vi "GUI_DS-LaserFrontEndLogger.vi"() -> ()   [LabVIEW 2013]
uses:
  Shared/GUI_Template/GUI_master/tcp_new_data_event.ctl
  Shared/GUI_Template/GUI_master/tcp new data cluster.ctl
panel:
  out "XY Graph 3":cluster{timestamp[], dbl[]}[](graph)
  out "XY Graph 2":cluster{timestamp[], dbl[]}[](graph)
  out "XY Graph":cluster{timestamp[], dbl[]}(graph)
  in  "reading.var 7::1":dbl caption="Preamp1 power" min=-100000.0 max=100000.0
  in  "reading.var 6::1":dbl caption="Amp0 pulse energy" min=-100000.0 max=100000.0
  in  "reading.var 1::1":dbl caption="Regen pulse energy" min=-100000.0 max=100000.0
  in  "reading.var 3::1":dbl caption="XPW spectral width" min=-100000.0 max=100000.0
  in  "reading.var 2::1":dbl caption="XPW spec peak counts" min=-100000.0 max=100000.0
  out "tcp data event":T1
  in  "Refresh Button":bool
  out "XY Graph 5":T2(graph)
  in  "channel 2::2":dbl[](array[numeric]) caption="channel 1::2"
  in  "GUIdevice 2":string="DS-XPWspec"
  in  "channel 1::2":dbl[](array[numeric])
  in  "reading.var 8::1":dbl caption="XPW central wavelength" min=-100000.0 max=100000.0
  in  "refresh time (ms)":i32=500
  in  "reading.var 5::1":dbl caption="Amp0 input centriod Y" min=-100000.0 max=100000.0
  in  "reading.var 4::1":dbl caption="Amp0 input centriod x" min=-100000.0 max=100000.0
  in  "stop":bool
  in  "GUIdevice 1":string="DS-LaserFrontEndLogger"
  # "Laser front end logger"
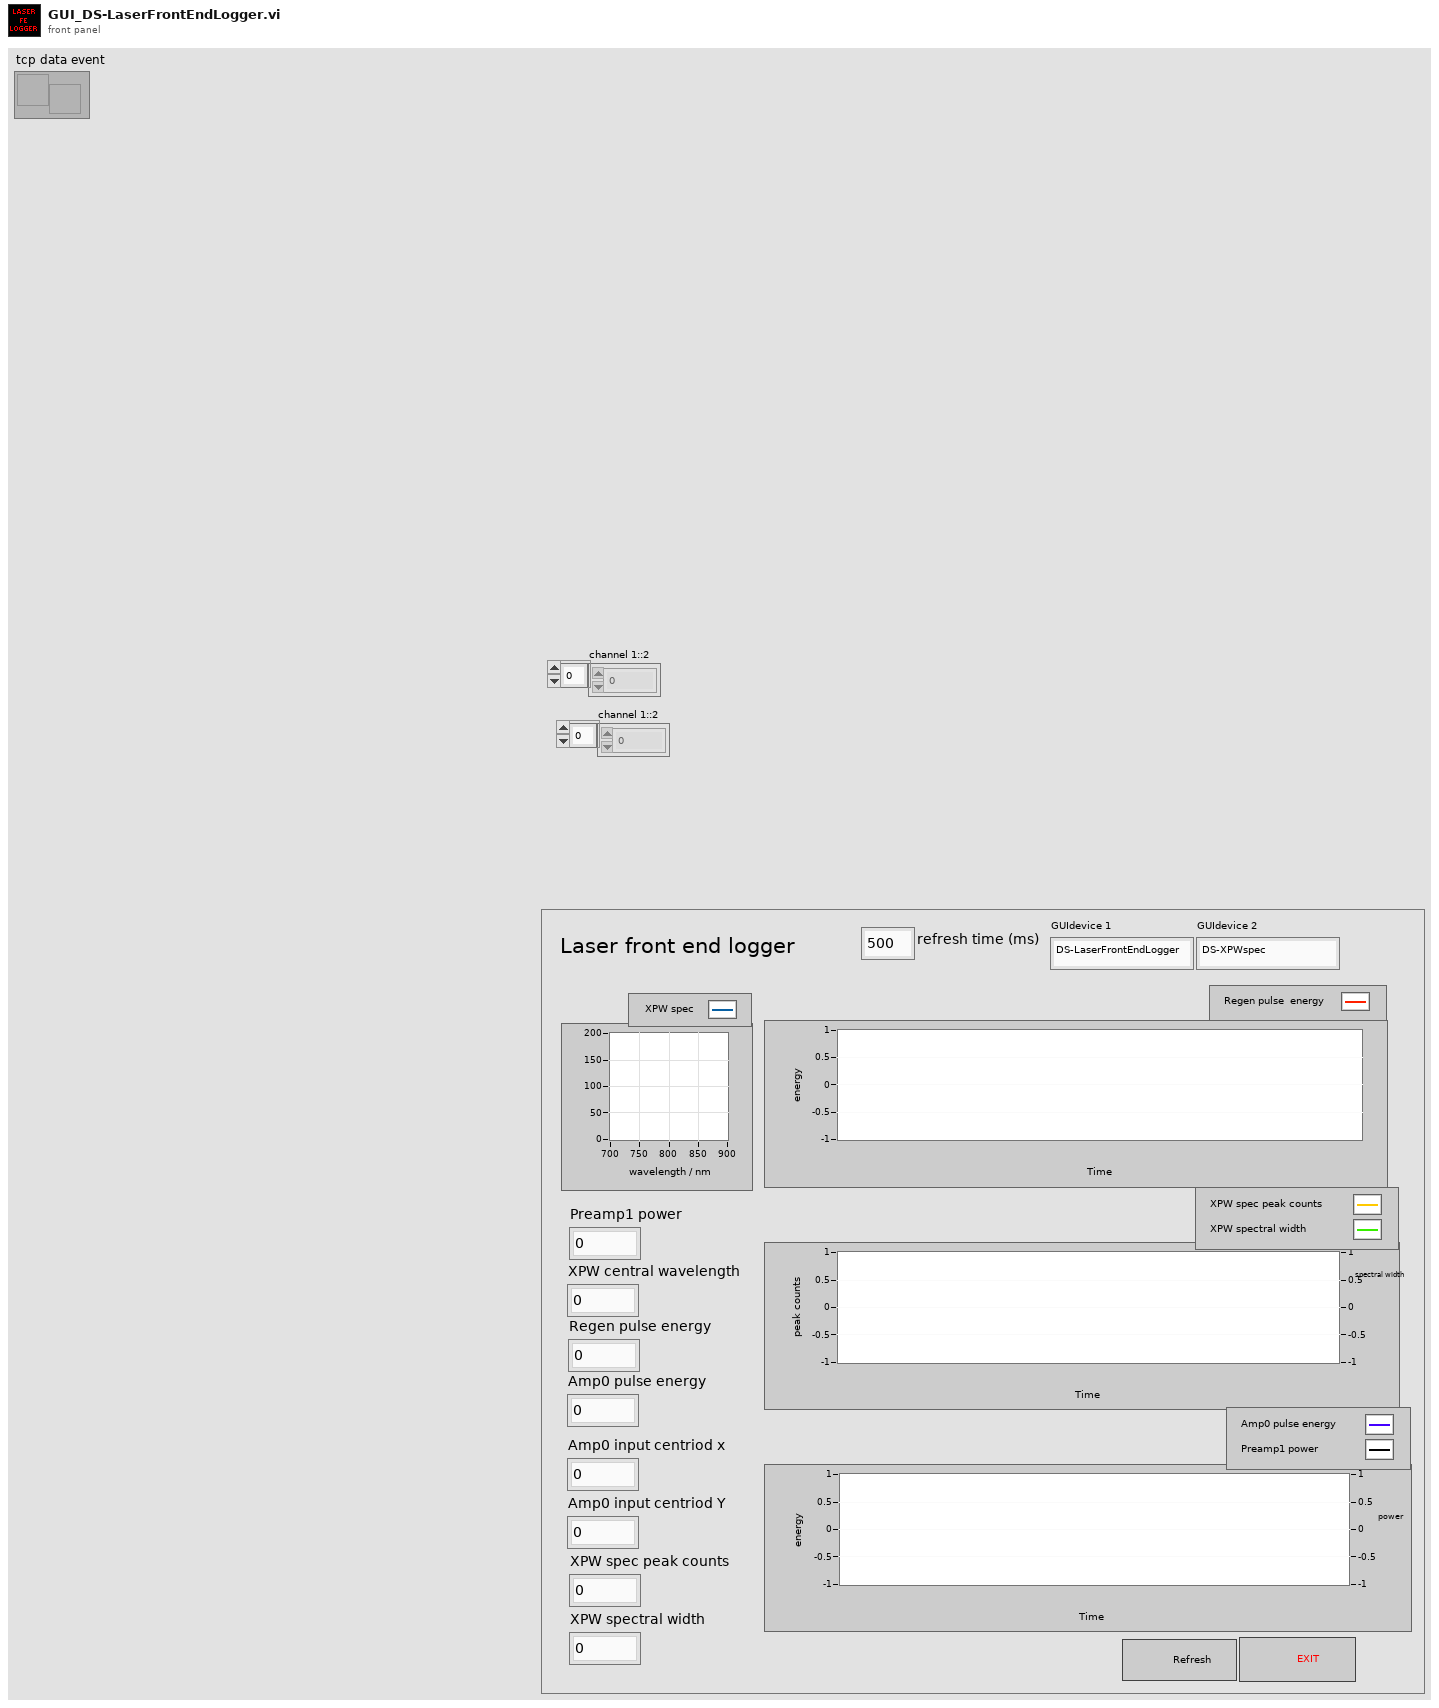
[diagram p1: front panel]
types:
  T1 = typedef "tcp_new_data_event.ctl" = refnum<user-event>
  T2 = cluster{"channel 1::2":dbl[], "channel 2::2":dbl[]}
  T3 = enum32{"invalid app kind", "Development System", "Run Time System", "Student Edition", "Embedded LabVIEW", "Evaluation", "Custom"}
  T4 = typedef "tcp new data cluster.ctl" = cluster{"EventEnum":enum16{"new data", "connection status update"}, "Device name":string}
  T5 = enum32{"Invalid", "Standard", "Closed", "Hidden", "Minimized", "Maximized"}
  T6 = cluster{"Core":cluster{"Current VI Reference":refnum<vi>, "Close Panel on Exit?":bool}, "Your Boolean data":bool, "Your string data":string, "SuperGUI":cluster{"STOP queue":refnum<queue>, "SuperGUI ref":refnum<vi>}, "Graph parameters":cluster{"Timestamp":dbl[], "variable 1":dbl[], "variable 2":dbl[], "variable 3":dbl[], "variable 7":dbl[], "variable 8":dbl[]}}
  T7 = cluster{"Timestamp":dbl[], "variable 1":dbl[], "variable 2":dbl[], "variable 3":dbl[], "variable 7":dbl[], "variable 8":dbl[]}
  T8 = cluster{"STOP queue":refnum<queue>, "SuperGUI ref":refnum<vi>}
  T9 = cluster{"Current VI Reference":refnum<vi>, "Close Panel on Exit?":bool}
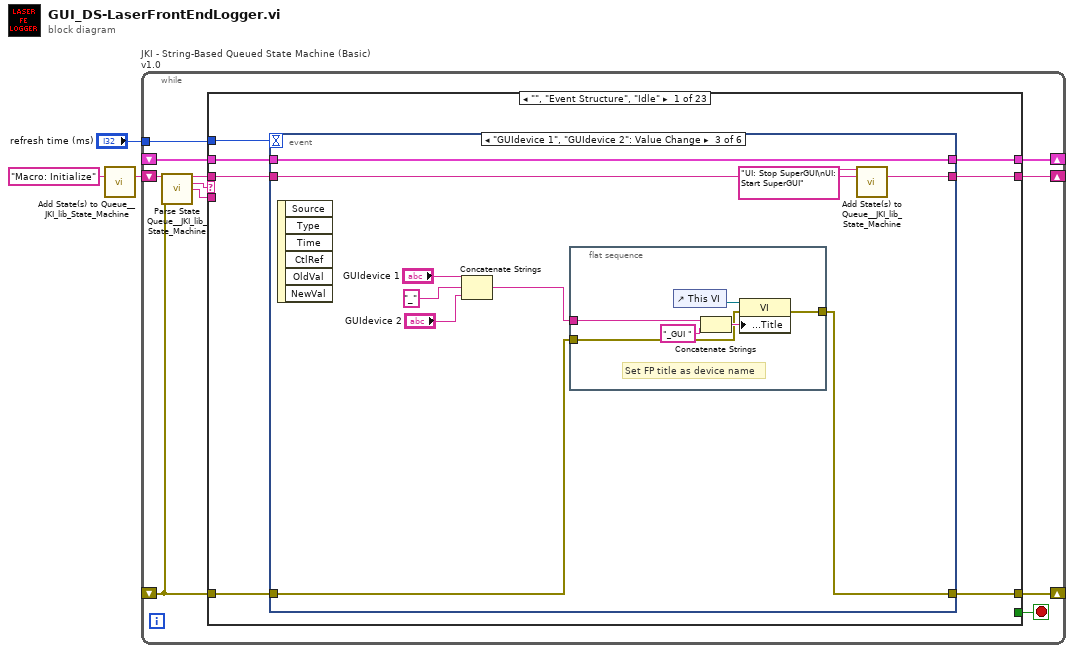
[diagram p0: block diagram]
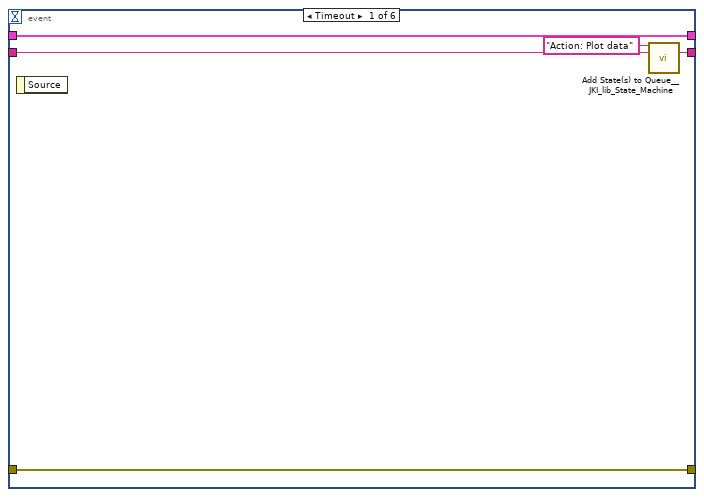
[diagram p2: hidden frame]
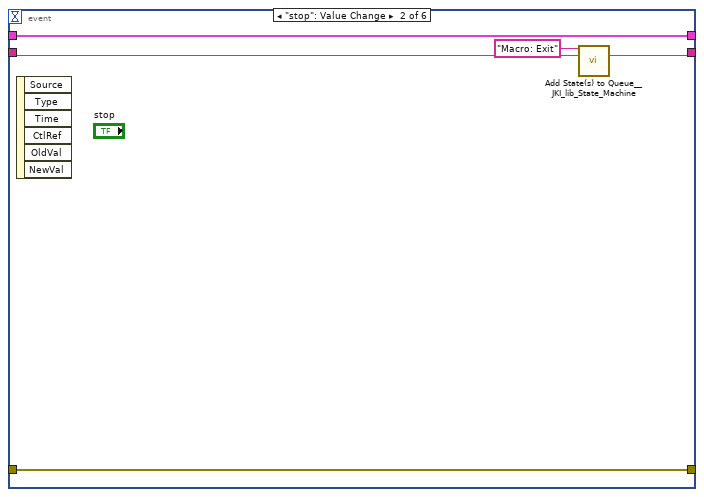
[diagram p3: hidden frame]
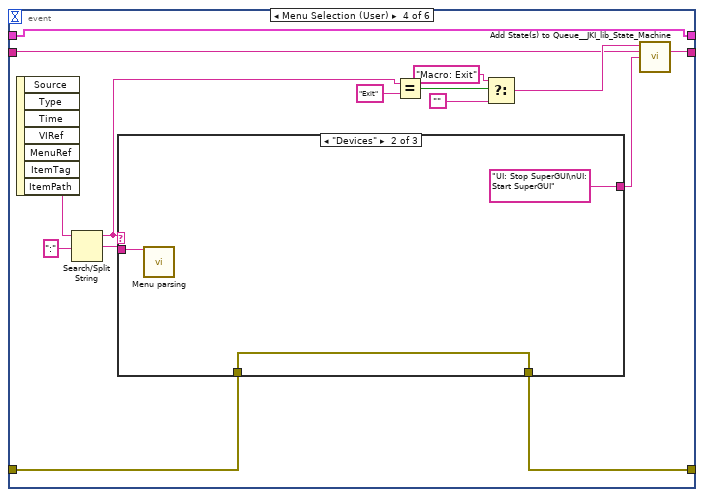
[diagram p4: hidden frame]
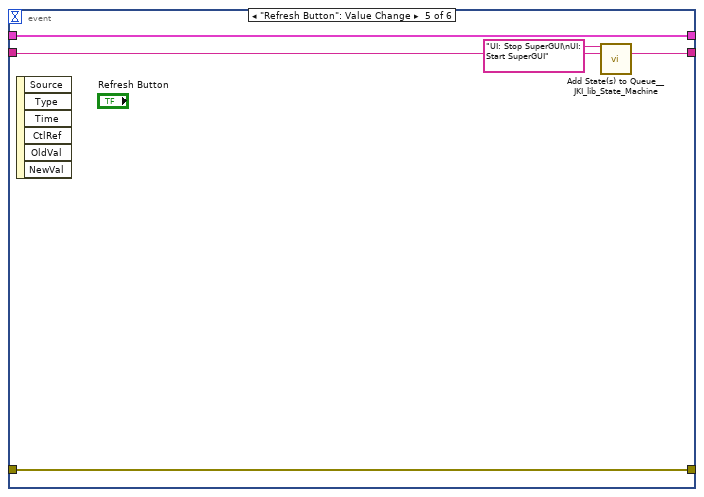
[diagram p7: hidden frame]
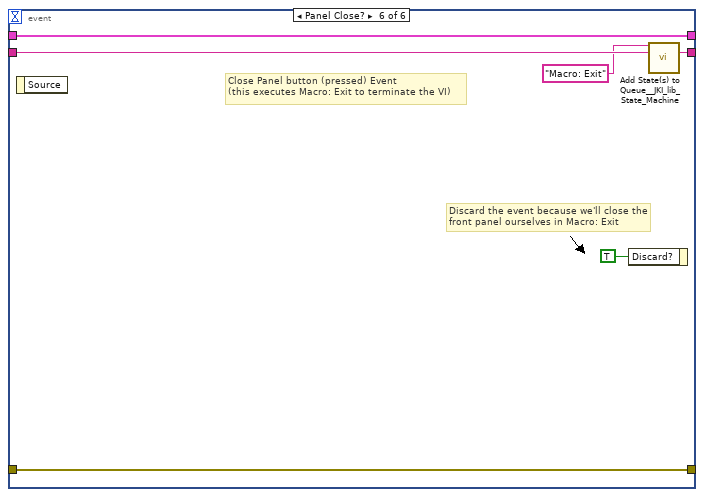
[diagram p8: hidden frame]
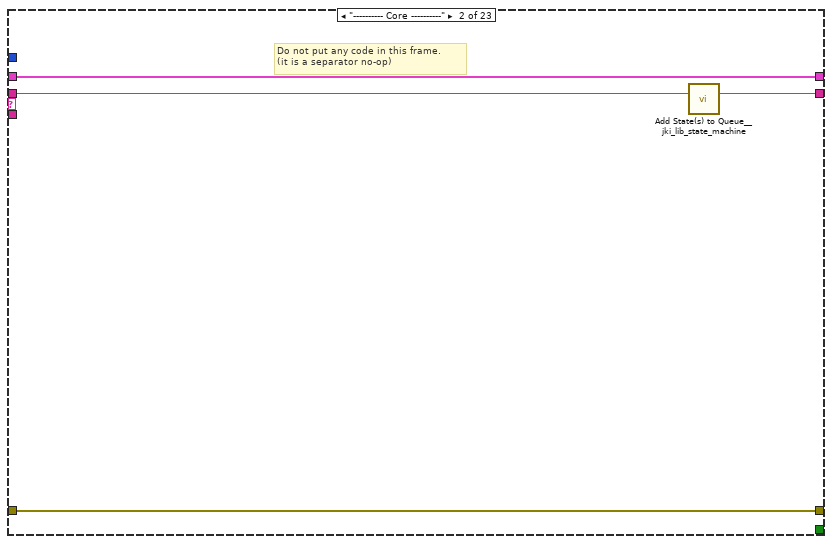
[diagram p9: hidden frame]
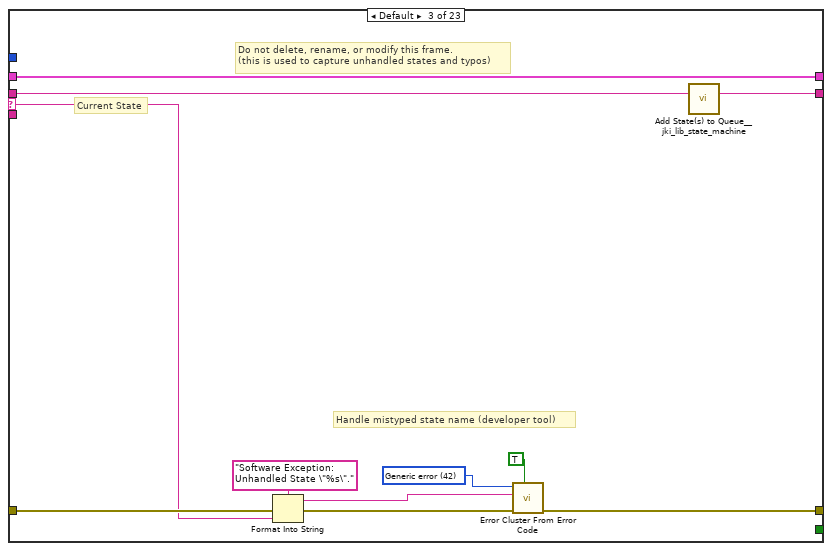
[diagram p10: hidden frame]
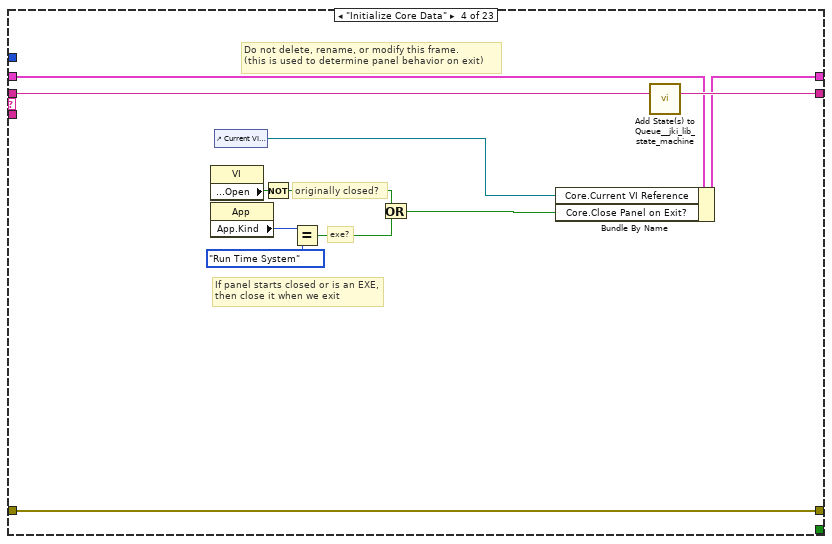
[diagram p11: hidden frame]
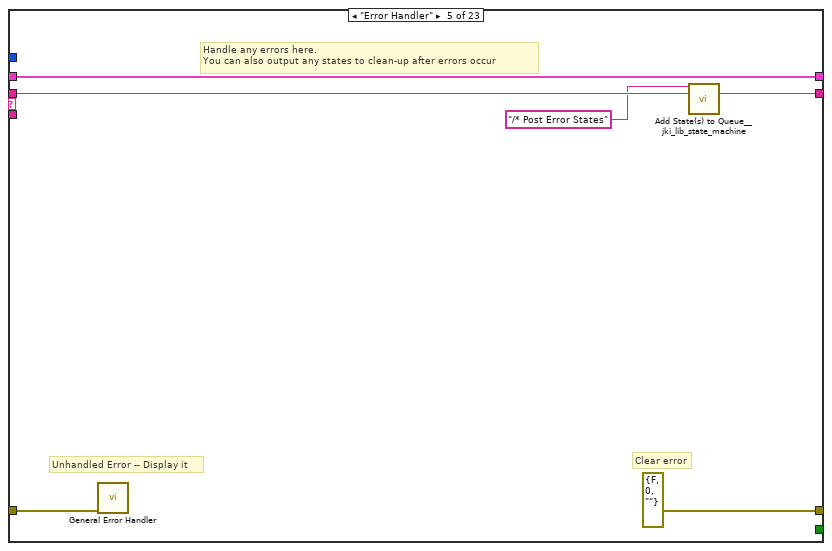
[diagram p12: hidden frame]
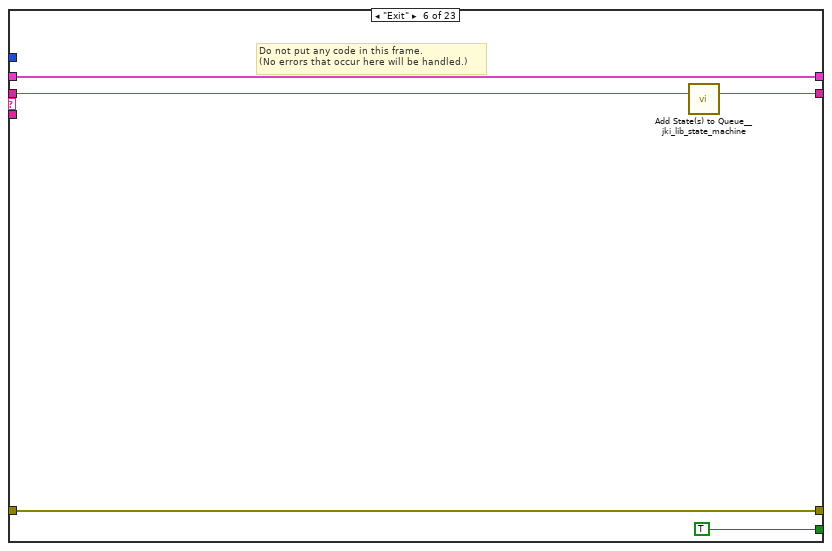
[diagram p13: hidden frame]
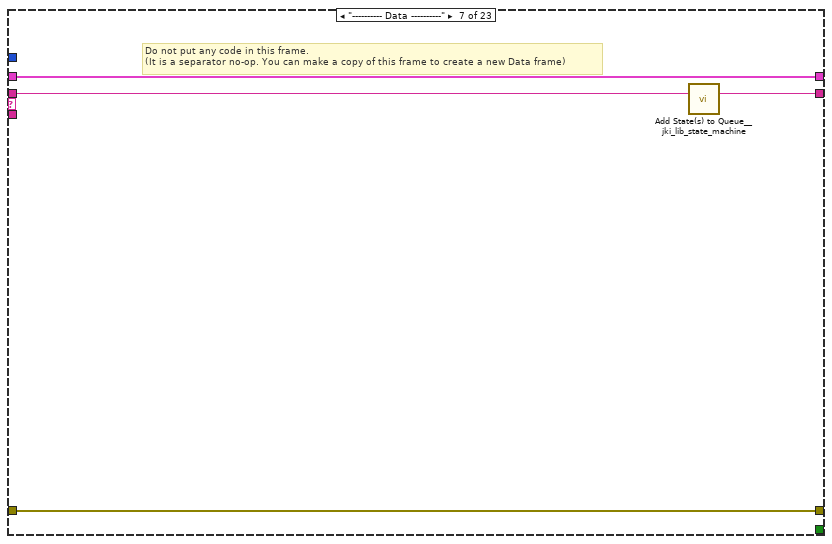
[diagram p14: hidden frame]
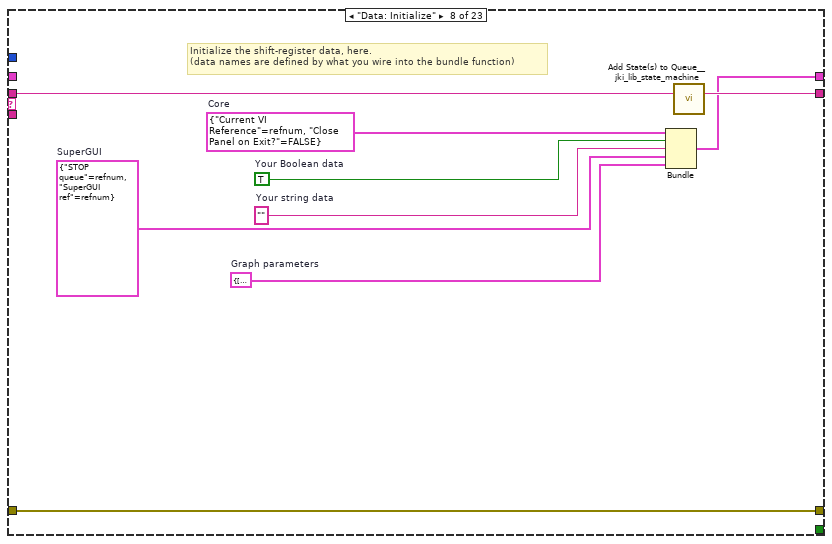
[diagram p15: hidden frame]
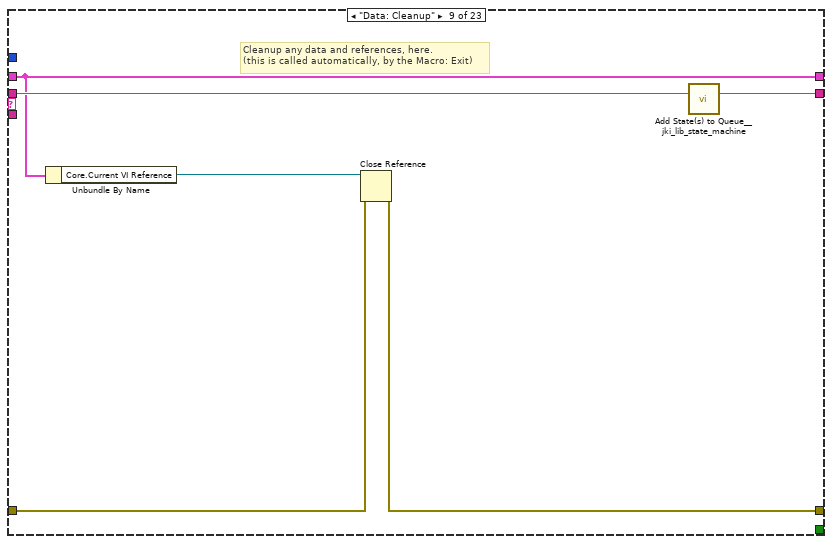
[diagram p16: hidden frame]
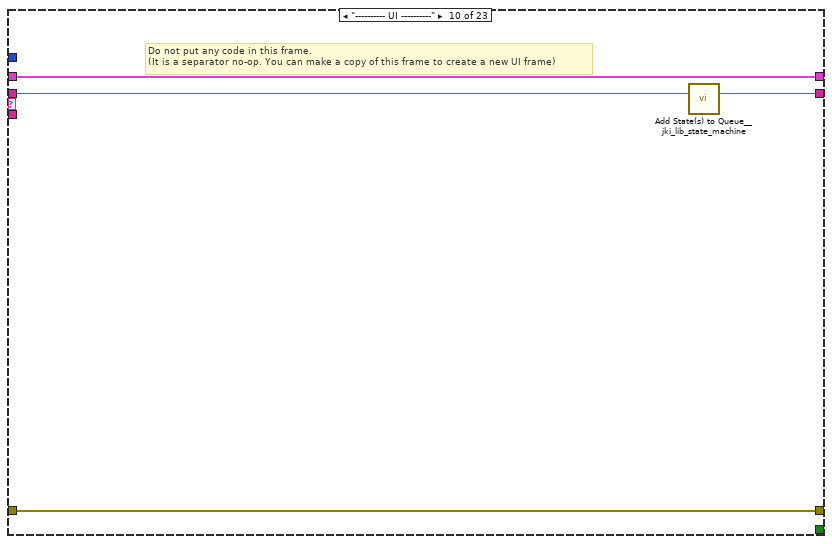
[diagram p17: hidden frame]
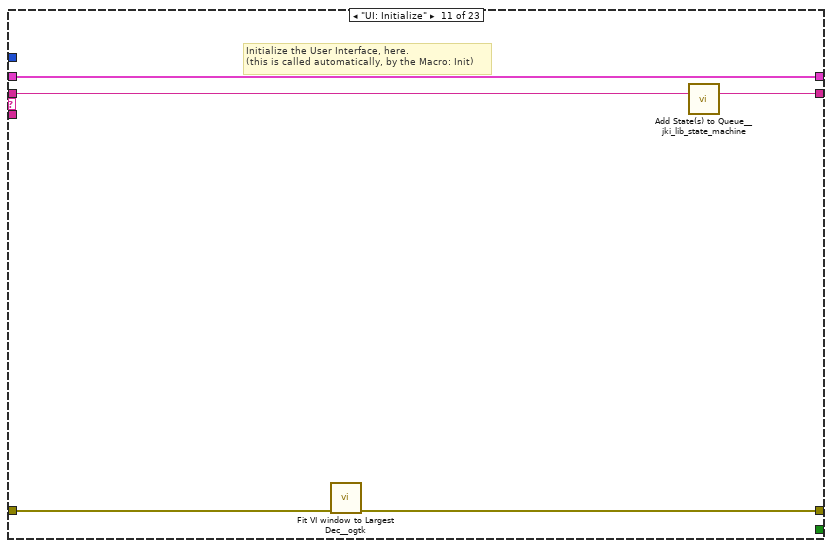
[diagram p18: hidden frame]
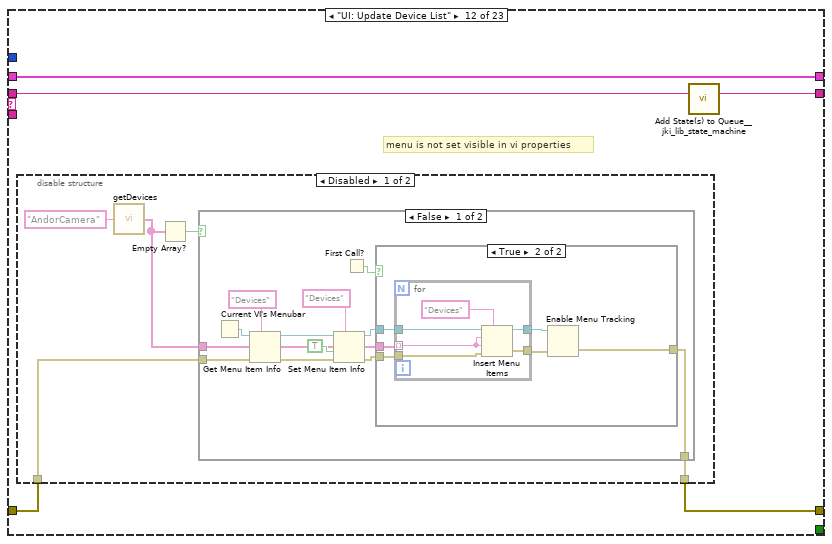
[diagram p19: hidden frame]
diagram:
  n1 = call <vilib>:"Add State(s) to Queue__JKI_lib_State_Machine.vi"("State(s) in (\"\")"="Macro: Initialize") -> ("States Out"=w3:string)  [unwired: 14 in]
  n2 = while "JKI - String-Based Queued State Machine (Basic) v1.0" {
    shift-right: [w7] -> _
    shift-left: _ -> [w6]
    shift-right: [w10] -> _
    shift-left: _ -> [w5]
    shift-right: [w9] -> _
    shift-left: w3 -> [w11]
    tunnel: "refresh time (ms)" -> [w4]
    stop <- w8 stop-if-true
    n3 = call <vilib>:"Parse State Queue__JKI_lib_State_Machine.vi"("State Queue"=w11, "Error In (no error)"=w5) -> ("Remaining States"=w13:string, "Current State"=w14:string, "Arguments"=w12:string)  [unwired: 11 in]
    n4 = case shown="\"\", \"Event Structure\", \"Idle\"" w14 {
      selector: w14 -> [_ _ w83 _ _ _ _ _ _ _ _ _ _ _ _ _ _ _ _ _ _ _ _]
      tunnel: w13 -> [w21 w82 w87 w105 w111 w116 w120 w129 w135 w139 w144 w149 w187 w221 w229 w235 w246 w272 w277 w287 w291 w329 w376]
      tunnel: w12 -> [_ _ _ _ _ _ _ _ _ _ _ _ _ _ _ w230 w240 _ _ _ _ _ _]
      tunnel: w6 -> [w19 w79 w85 w96 w108 w114 w117 _ w130 w136 w142 w147 w185 w212 w224 w233 w242 w269 w274 w284 w288 w299 w373]
      tunnel: [w18 w80 w89 w102 errorcluster {"status"=FALSE, "code"=0, "source"=""} ("error out") w113 w118 w126 w131 w137 w140 w145 w182 w205 w222 w231 w243 w270 w275 w285 w289 w327 w374] -> w10
      tunnel: w5 -> [w17 w80 w88 w102 w107 w113 w118 w126 w132 w137 w141 w146 w183 w206 w223 w232 w244 w270 w275 w285 w289 w327 w374]
      tunnel: [w20 w81 w86 w104 w110 w115 w119 w128 w134 w138 w143 w148 w186 w220 w228 w234 w245 w271 w276 w286 w290 w328 w375] -> w9
      tunnel: [_ _ _ _ _ TRUE _ _ _ _ _ _ _ _ _ _ _ _ _ _ _ _ _] -> w8
      tunnel: [w16 w79 w85 w103 w108 w114 w117 w127 w130 w136 w142 w147 w185 w211 w224 w233 w242 w269 w274 w284 w288 w298 w373] -> w7
      tunnel: w4 -> [w15 _ _ _ _ _ _ _ _ _ _ _ _ _ _ _ _ _ _ _ _ _ _]
      frame "", "Event Structure", "Idle" {
        n5 = event shown="[2] \"GUIdevice 1\", \"GUIdevice 2\": Value Change" {
          selector: _ -> [_ _ _ _ _ _]
          dyn-events: _ -> [_ _ _ _ _ _]
          timeout: w15 -> [_ _ _ _ _ _]
          tunnel: w21 -> [w26 w29 w40 w56 w70 w78]
          tunnel: [w25 w28 w39 w55 w69 w77] -> w20
          tunnel: w19 -> [w23 w31 w41 w62 w72 w75]
          tunnel: [w24 w30 w33 w49 w71 w76] -> w18
          tunnel: w17 -> [w24 w30 w34 w50 w71 w76]
          tunnel: [w23 w31 w41 w62 w72 w75] -> w16
          event Timeout {
            n6 = event-data() -> ()  [unwired: 1 in, 1 out]
            n7 = call <vilib>:"Add State(s) to Queue__JKI_lib_State_Machine.vi"("State(s) in Front (\"\")"="Action: Plot data" ("State(s) in Front (\"\")"), "State(s) in (\"\")"=w26) -> ("States Out"=w25:string)  [unwired: 13 in]
          }
          event "stop": Value Change {
            n8 = event-data() -> ()  [unwired: 1 in, 6 out]
            n9 = call <vilib>:"Add State(s) to Queue__JKI_lib_State_Machine.vi"("State(s) in Front (\"\")"="Macro: Exit", "State(s) in (\"\")"=w29) -> ("States Out"=w28:string)  [unwired: 13 in]
          }
          event "GUIdevice 1", "GUIdevice 2": Value Change {
            n10 = event-data() -> ()  [unwired: 1 in, 6 out]
            n11 = Concatenate Strings("GUIdevice 1", "_", "GUIdevice 2") -> (w35:string)
            n12 = flat-sequence {
              tunnel: [w44] -> w33
              tunnel: w34 -> [w43]
              tunnel: w35 -> [w42]
              frame #0 {
                # "Set FP title as device name"
                n13 = control-ref of="This VI"() -> (w47:refnum<vi>)
                n14 = Concatenate Strings(w42, "_GUI ") -> (w46:string)
                n15 = property class="VI"(reference=w47, error in=w43, "Front Panel.Title"=w46) -> (error out=w44:errorcluster)  [unwired: 1 out]
              }
            }
            n16 = call <vilib>:"Add State(s) to Queue__JKI_lib_State_Machine.vi"("State(s) in Front (\"\")"="UI: Stop SuperGUI\nUI: Start SuperGUI", "State(s) in (\"\")"=w40) -> ("States Out"=w39:string)  [unwired: 13 in]
          }
          event Menu Selection (User) {
            n17 = event-data() -> ("ItemPath"=w52:string)  [unwired: 1 in, 6 out]
            n18 = Search/Split String(string=w52, search string/char (-)=":") -> (substring before match=w48:string, match + rest of string=w51:string)  [unwired: 1 in, 1 out]
            n19 = case shown="\"Devices\"" w48 {
              tunnel: w51 -> [_ w66 _]
              tunnel: w50 -> [w63 w64 w67]
              tunnel: [w63 w64 w67] -> w49
              tunnel: [_ "UI: Stop SuperGUI\nUI: Start SuperGUI" _] -> w54
              frame "", Default {
              }
              frame "Devices" {
                n20 = call "Menu parsing.vi"("ItemPath"=w66) -> ()  [unwired: 9 in, 2 out]
              }
              frame "Exit" {
              }
            }
            n21 = Equal?(x=w48, y="Exit") -> (x = y?=w60:bool)
            n22 = Select(t="Macro: Exit", s=w60, f="") -> (s? t:f=w57:string)
            n23 = call <vilib>:"Add State(s) to Queue__JKI_lib_State_Machine.vi"("State(s) in Front (\"\")"=w57, "State(s) in (\"\")"=w56, "State(s) at Back (\"\")"=w54) -> ("States Out"=w55:string)  [unwired: 12 in]
          }
          event "Refresh Button": Value Change {
            n24 = event-data() -> ()  [unwired: 1 in, 6 out]
            n25 = call <vilib>:"Add State(s) to Queue__JKI_lib_State_Machine.vi"("State(s) in Front (\"\")"="UI: Stop SuperGUI\nUI: Start SuperGUI", "State(s) in (\"\")"=w70) -> ("States Out"=w69:string)  [unwired: 13 in]
          }
          event Panel Close? {
            # "Discard the event because we'll close the front panel ourselves in Macro: Exit"
            # "Close Panel button (pressed) Event\n(this executes Macro: Exit to terminate the VI)"
            n26 = event-data() -> ()  [unwired: 1 in, 1 out]
            n27 = event-data("Discard?"=TRUE) -> ()  [unwired: 1 in, 1 out]
            n28 = call <vilib>:"Add State(s) to Queue__JKI_lib_State_Machine.vi"("State(s) in Front (\"\")"="Macro: Exit", "State(s) in (\"\")"=w78) -> ("States Out"=w77:string)  [unwired: 13 in]
          }
        }
      }
      frame "---------- Core ----------" {
        # "Do not put any code in this frame.\n(it is a separator no-op)"
        n29 = call <vilib>:"Add State(s) to Queue__jki_lib_state_machine.vi"("State(s) in (\"\")"=w82) -> ("States Out"=w81:string)  [unwired: 14 in]
      }
      frame Default {
        w92 = 42 items=["No error", "Argument error", "Memory is full", "Out of zone", "End of file", "File already open", "Generic file I/O error", "File not found", "File permission error", "Disk is full", "Duplicate path", "Too many files open", "System feature not enabled", "Resource file not found", "Cannot add resource", "Resource not found", "Image not found", "Image memory error", "Pen does not exist", "Config type invalid", "Config token not found", "Config parse error", "Config memory error", "Bad external code format", "Bad external code offset", "External code not present", "Null window", "Destroy window error", "Null menu", "Print aborted", "Bad print record", "Print driver error", "Windows error during printing", "Memory error during printing", "Print dialog error", "Generic print error", "Invalid device refnum", "Device not found", "Device parameter error", "Device unit error", "Cannot open device", "Device call aborted", "Generic error", "Cancelled by user", "Object ID too low", "Object ID too high", "Object not in heap", "Unknown heap", "Unknown object (invalid DefProc)", "Unknown object (DefProc not in table)", "Message out of range", "Invalid (null) method", "Unknown message", "Manager call not supported", "Bad address", "Network operation in progress", "Network operation timed out", "Connection is busy", "Network attribute not supported", "Network error", "Address in use", "System out of memory", "Connection aborted", "Connection refused", "Not connected", "Already connected", "Connection closed", "Initialization error (interapplication manager)", "Bad occurrence", "Wait on unbound occurrence handler", "Occurrence queue overflow", "Datalog type conflict", "Unused", "Unrecognized type (interapplication manager)", "Memory corrupt", "Failed to make temporary DLL", "Old CIN version", "Drag socket not found", "Failed to load drop-object", "Failed to register OLE object", "Failed to release OLE object", "Format specifier type mismatch", "Unknown format specifier", "Too few format specifiers", "Too many format specifiers", "Scan failed", "Newer CIN version", "Error converting to variant", "Runtime menu error", "Password tampered", "Variant attribute not found", "Incompatible variant data type", "Event data is not available", "Event Store is not present", "Occurrence is not found", "Event Queue is not created", "Event info is not available", "Refnum passed is NULL", "Error retrieving Class GUID", "Error retrieving CoClass GUID", "Error retrieving TypeLib GUID.", "Bad built application magic bytes.", "Specific driver is different from the specific driver associated with the Logical Name.", "There is no session opened to the class driver.", "Max Error", "MAX - Error with config objects", "MAX - Error loading configuration", "MAX - Group not supported"]
        # "Current State"
        # "Do not delete, rename, or modify this frame.\n(this is used to capture unhandled states and typos)"
        # "Handle mistyped state name (developer tool)"
        n30 = Format Into String(format string="Software Exception: Unhandled State \"%s\"." ("message"), error in=w88, w83) -> (resulting string=w91:string, error out=w90:errorcluster)  [unwired: 1 in]
        n31 = call <vilib>:"Error Cluster From Error Code.vi"("show call chain? (False)"=TRUE, "error in (no error)"=w90, "error message (\"\")"=w91, "error code (0)"=w92) -> ("error out"=w89:errorcluster)  [unwired: 5 in]
        n32 = call <vilib>:"Add State(s) to Queue__jki_lib_state_machine.vi"("State(s) in (\"\")"=w87) -> ("States Out"=w86:string)  [unwired: 14 in]
      }
      frame "Initialize Core Data" {
        # "Do not delete, rename, or modify this frame.\n(this is used to determine panel behavior on exit)"
        # "originally closed?"
        # "exe?"
        # "If panel starts closed or is an EXE, then close it when we exit"
        n33 = property class="VI"() -> ("Front Panel.Open"=w101:bool)  [unwired: 2 in, 2 out]
        n34 = property class="App"() -> ("App.Kind"=w100:T3)  [unwired: 2 in, 2 out]
        n35 = control-ref of="Current VI Reference"() -> (w94:refnum<vi>)
        n36 = Not(x=w101) -> (.not. x?=w98:bool)
        n37 = Equal?(x=w100, y=T3."Run Time System" ("Application:Kind")) -> (x = y?=w97:bool)
        n38 = Or(x=w98, y=w97) -> (x .or. y?=w95:bool)
        n39 = Bundle By Name(cluster=w96, "Core.Current VI Reference"=w94, "Core.Close Panel on Exit?"=w95) -> (w103:T6)
        n40 = call <vilib>:"Add State(s) to Queue__jki_lib_state_machine.vi"("State(s) in (\"\")"=w105) -> ("States Out"=w104:string)  [unwired: 14 in]
      }
      frame "Error Handler" {
        # "Unhandled Error -- Display it"
        # "Handle any errors here.\nYou can also output any states to clean-up after errors occur"
        # "Clear error"
        n41 = call <vilib>:"General Error Handler.vi"("error in (no error)"=w107) -> ()  [unwired: 10 in, 5 out]
        n42 = call <vilib>:"Add State(s) to Queue__jki_lib_state_machine.vi"("State(s) in Front (\"\")"="/* Post Error States", "State(s) in (\"\")"=w111) -> ("States Out"=w110:string)  [unwired: 13 in]
      }
      frame "Exit" {
        # "Do not put any code in this frame.\n(No errors that occur here will be handled.)"
        n43 = call <vilib>:"Add State(s) to Queue__jki_lib_state_machine.vi"("State(s) in (\"\")"=w116) -> ("States Out"=w115:string)  [unwired: 14 in]
      }
      frame "---------- Data ----------" {
        # "Do not put any code in this frame.\n(It is a separator no-op. You can make a copy of this frame to create a new Data frame)"
        n44 = call <vilib>:"Add State(s) to Queue__jki_lib_state_machine.vi"("State(s) in (\"\")"=w120) -> ("States Out"=w119:string)  [unwired: 14 in]
      }
      frame "Data: Initialize" {
        w121 = T7 {"Timestamp"=[], "variable 1"=[], "variable 2"=[], "variable 3"=[], "variable 7"=[], "variable 8"=[]}  # Graph parameters
        w122 = T8 {"STOP queue"=refnum, "SuperGUI ref"=refnum}  # SuperGUI
        w123 = T9 {"Current VI Reference"=refnum, "Close Panel on Exit?"=FALSE}  # Core
        w125 = TRUE  # Your Boolean data
        w124 = ""  # Your string data
        # "Initialize the shift-register data, here.\n(data names are defined by what you wire into the bundle function)"
        n45 = Bundle("Core"=w123, "Your Boolean data"=w125, "Your string data"=w124, "SuperGUI"=w122, "Graph parameters"=w121) -> (w127:T6)  [unwired: 1 in]
        n46 = call <vilib>:"Add State(s) to Queue__jki_lib_state_machine.vi"("State(s) in (\"\")"=w129) -> ("States Out"=w128:string)  [unwired: 14 in]
      }
      frame "Data: Cleanup" {
        # "Cleanup any data and references, here.\n(this is called automatically, by the Macro: Exit)"
        n47 = Unbundle By Name(w130) -> ("Core.Current VI Reference"=w133:refnum<vi>)
        n48 = Close Reference(reference=w133, error in (no error)=w132) -> (error out=w131:errorcluster)
        n49 = call <vilib>:"Add State(s) to Queue__jki_lib_state_machine.vi"("State(s) in (\"\")"=w135) -> ("States Out"=w134:string)  [unwired: 14 in]
      }
      frame "---------- UI ----------" {
        # "Do not put any code in this frame.\n(It is a separator no-op. You can make a copy of this frame to create a new UI frame)"
        n50 = call <vilib>:"Add State(s) to Queue__jki_lib_state_machine.vi"("State(s) in (\"\")"=w139) -> ("States Out"=w138:string)  [unwired: 14 in]
      }
      frame "UI: Initialize" {
        # "Initialize the User Interface, here.\n(this is called automatically, by the Macro: Init)"
        n51 = call <userlib>:"Fit VI window to Largest Dec__ogtk.vi"("error in (no error)"=w141) -> ("error out"=w140:errorcluster)  [unwired: 5 in, 1 out]
        n52 = call <vilib>:"Add State(s) to Queue__jki_lib_state_machine.vi"("State(s) in (\"\")"=w144) -> ("States Out"=w143:string)  [unwired: 14 in]
      }
      frame "UI: Update Device List" {
        # "menu is not set visible in vi properties"
        n53 = disable-structure shown="Disabled" {
          disable-tunnel: w146 -> [w154 w181]
          disable-tunnel: [w152 w181] -> w145
          frame Disabled {
            n54 = call "getDevices.vi"("Device Class"="AndorCamera") -> ("All Devices"=w150:string[])
            n55 = Empty Array?(array=w150) -> (empty?=w151:bool)
            n56 = case shown="False" w151 {
              tunnel: w154 -> [w157 w180]
              tunnel: [w156 w180] -> w152
              tunnel: w150 -> [w155 _]
              frame False {
                n57 = Current VI's Menubar() -> (w160:refnum<k9>)
                n58 = Get Menu Item Info(7:"Devices" ("item tag"), 8:w157, 11:w160) -> (0:w166:errorcluster, 3:w162:refnum<k9>)  [unwired: 5 out]
                n59 = Set Menu Item Info(7:"Devices" ("item tag"), 8:w166, 9:TRUE ("enabled"), 11:w162) -> (0:w165:errorcluster, 3:w164:refnum<k9>)  [unwired: 3 in]
                n60 = First Call?() -> (First Call?: T/F=w158:bool)
                n61 = case shown="True" w158 {
                  tunnel: w164 -> [_ w172]
                  tunnel: w155 -> [_ w171]
                  tunnel: w165 -> [w167 w169]
                  tunnel: [w167 w168] -> w156
                  frame False {
                  }
                  frame True {
                    n62 = for {
                      tunnel: [w179] -> w173
                      tunnel: w171 -> [w177] mode=indexing
                      tunnel: w172 -> [w176]
                      tunnel: [w175] -> w170
                      tunnel: w169 -> [w174]
                      n63 = Insert Menu Items(5:"Devices" ("menu tag"), 6:w174, 7:w177, 8:w177, 9:w176) -> (0:w175:errorcluster, 3:w179:refnum<k9>)  [unwired: 1 in, 1 out]
                    }
                    n64 = Enable Menu Tracking(2:w170, 4:w173) -> (0:w168:errorcluster)  [unwired: 1 in, 1 out]
                  }
                }
              }
              frame True {
              }
            }
          }
          frame Enabled {
          }
        }
        n65 = call <vilib>:"Add State(s) to Queue__jki_lib_state_machine.vi"("State(s) in (\"\")"=w149) -> ("States Out"=w148:string)  [unwired: 14 in]
      }
      frame "UI: Get Device Name" {
        n66 = First Call?() -> (First Call?: T/F=w184:bool)
        n67 = case shown="True" w184 {
          tunnel: w183 -> [w188 w190]
          tunnel: [w188 w189] -> w182
          frame False {
          }
          frame True {
            n68 = disable-structure "Get Device name from control for vi mode\nand command line arg for exe" shown="RUN_TIME_ENGINE==True" {
              disable-tunnel: w190 -> [w191 w193]
              disable-tunnel: [w191 w192] -> w189
              frame condition #0 (active) {
              }
              frame condition #1 {
                n69 = control-ref of="This Application"() -> (w201:refnum<vi>)
                n70 = property class="App"(reference=w201) -> ("App.Args"=w200:string[])  [unwired: 1 in, 2 out]
                n71 = Index Array(array=w200, index #1=1 ("index")) -> (element #1=w194:string)  [unwired: 2 in, 2 out]
                n72 = Empty String/Path?(string/path=w194) -> (empty?=w198:bool)
                n73 = control-ref of="This VI"() -> (w197:refnum<vi>)
                n74 = case shown="False" w198 {
                  frame False {
                  }
                  frame True {
                  }
                }
                n75 = Concatenate Strings(w194, "_GUI ") -> (w196:string)
                n76 = property class="VI"(reference=w197, error in=w193, "Front Panel.Title"=w196) -> (error out=w192:errorcluster)  [unwired: 1 out]
              }
            }
          }
        }
        n77 = call <vilib>:"Add State(s) to Queue__jki_lib_state_machine.vi"("State(s) in (\"\")"=w187) -> ("States Out"=w186:string)  [unwired: 14 in]
      }
      frame "UI: Start SuperGUI" {
        # "create stop queue for supergui and its clones"
        # "x100 abort will be dependent on caller VI\nx80 abort will be independent of caller vi, this will abort vi when labview is closed."
        # "Start SuperGUI asynchronous way"
        n78 = vi-ref "GUI_Master_subvi_reentrant_queues.vi"() -> (w204:refnum<vi>)
        n79 = property class="VI"(reference=w204) -> ("Path"=w203:path)  [unwired: 1 in, 2 out]
        n80 = Create User Event(user event datatype=T4 {"EventEnum"=enum."new data", "Device name"="Device name"} ("New Event"), error in=w206) -> (user event=w207:refnum<user-event>, error out=w213:errorcluster)
        "tcp data event" <- w207
        n81 = control-ref of="This Application"() -> (w210:refnum<vi>)
        n82 = control-ref of="This VI"() -> (w209:refnum<vi>)
        n83 = Open VI Reference(type specifier VI Refnum (for type only)=refnum<vi> refnum, vi path=w203, options=256) -> (vi reference=w219:refnum<vi>, error out=w218:errorcluster)  [unwired: 3 in]
        n84 = register-events(w207) -> ()  [unwired: 2 in, 2 out]
        n85 = call "supergui create stop queue.vi"() -> ("STOP Queue out"=w215:refnum<queue>)  [unwired: 11 in]
        n86 = Current VI's Menubar() -> (w208:refnum<k9>)
        n87 = call-by-ref "Start Asynchronous Call"(reference=w219, error in=w218, "STOP Queue in"=w215, "This Application"=w210, 8:"error in (no error)"=w213, "tcp data event"=w207, "Caller menu reference"=w208, "Caller VI ref"=w209) -> (reference out=w202:refnum<vi>, error out=w205:errorcluster)  [unwired: 5 in, 1 out]
        n88 = Bundle By Name(cluster=w212, "SuperGUI.SuperGUI ref"=w202, "SuperGUI.STOP queue"=w215) -> (w211:T6)
        n89 = call <vilib>:"Add State(s) to Queue__jki_lib_state_machine.vi"("State(s) in (\"\")"=w221) -> ("States Out"=w220:string)  [unwired: 14 in]
      }
      frame "UI: Stop SuperGUI" {
        # "Stop Supergui Clone and wait until it exit properly"
        n90 = Unbundle By Name(w224) -> ("SuperGUI.SuperGUI ref"=w226:refnum<vi>, "SuperGUI.STOP queue"=w225:refnum<queue>)
        n91 = Release Queue(queue=w225, error in (no error)=w223) -> (error out=w227:errorcluster)  [unwired: 1 in, 2 out]
        n92 = call-by-ref "Wait On Asynchronous Call"(reference=w226, error in=w227) -> ("error out"=w222:errorcluster)  [unwired: 11 in, 2 out]
        n93 = call <vilib>:"Add State(s) to Queue__jki_lib_state_machine.vi"("State(s) in (\"\")"=w229) -> ("States Out"=w228:string)  [unwired: 14 in]
      }
      frame "UI: Cursor Set" {
        # "Argument"
        # "Set and Unset Cursor Busy.\n(Usage: \"UI: Cursor Set >> Busy|Idle\")"
        n94 = case shown="\"Idle\", Default" w230 {
          tunnel: w232 -> [w237 w239]
          tunnel: [w236 w238] -> w231
          frame "Idle", Default {
            n95 = call <vilib>:"Unset Busy.vi"("error in (no error)"=w237) -> ("error out"=w236:errorcluster)  [unwired: 10 in]
          }
          frame "Busy" {
            n96 = call <vilib>:"Set Busy.vi"("error in (no error)"=w239) -> ("error out"=w238:errorcluster)  [unwired: 9 in, 1 out]
          }
        }
        n97 = call <vilib>:"Add State(s) to Queue__jki_lib_state_machine.vi"("State(s) in (\"\")"=w235) -> ("States Out"=w234:string)  [unwired: 14 in]
      }
      frame "UI: Front Panel State" {
        # "Argument"
        # "Set Front Panel Open or Closed\n(Usage: \"UI: Front Panel State >> Open|Close\")"
        n98 = Unbundle By Name(w242) -> ("Core.Current VI Reference"=w241:refnum<vi>)
        n99 = case shown="\"Close\"" w240 {
          tunnel: w244 -> [w250 w263]
          tunnel: [w252 w264] -> w243
          tunnel: w241 -> [w251 w261]
          frame "Open", Default {
            n100 = property class="VI"(reference=w251, error in=w250) -> (reference out=w248:refnum<vi>, error out=w249:errorcluster, "Front Panel.Open"=w247:bool)
            n101 = case shown="False" w247 {
              tunnel: [w255 w258] -> w252
              tunnel: w249 -> [w254 w258]
              tunnel: w248 -> [w253 _]
              frame False {
                n102 = invoke class="VI" method="FP.Open"(reference=w253, error in=w254, "Activate"=TRUE, "State"=T5."Standard") -> (error out=w255:errorcluster)  [unwired: 1 in, 4 out]
              }
              frame True {
              }
            }
          }
          frame "Close" {
            n103 = property class="VI"(reference=w261, error in=w263) -> (reference out=w260:refnum<vi>, error out=w262:errorcluster, "Front Panel.Open"=w259:bool)
            n104 = case shown="True" w259 {
              tunnel: [w265 w268] -> w264
              tunnel: w262 -> [w265 w267]
              tunnel: w260 -> [_ w266]
              frame False {
              }
              frame True {
                n105 = invoke class="VI" method="FP.Close"(reference=w266, error in=w267) -> (error out=w268:errorcluster)  [unwired: 1 in, 2 out]
              }
            }
          }
        }
        n106 = call <vilib>:"Add State(s) to Queue__jki_lib_state_machine.vi"("State(s) in (\"\")"=w246) -> ("States Out"=w245:string)  [unwired: 14 in]
      }
      frame "---------- Macro ----------" {
        # "Do not put any code in this frame.\n(It is a separator no-op. You can make a copy of this frame to create a new Macro frame)"
        n107 = call <vilib>:"Add State(s) to Queue__jki_lib_state_machine.vi"("State(s) in (\"\")"=w272) -> ("States Out"=w271:string)  [unwired: 14 in]
      }
      frame "Macro: Initialize" {
        # "Initialization Macro\n(This is called once, when the VI starts)"
        n108 = call <vilib>:"Add State(s) to Queue__jki_lib_state_machine.vi"("State(s) in Front (\"\")"="Data: Initialize\nInitialize Core Data\nUI: Initialize\nUI: Update Device List\nUI: Get Device Name\nUI: Start SuperGUI\nUI: Front Panel State >> Open", "State(s) in (\"\")"=w277) -> ("States Out"=w276:string)  [unwired: 13 in]
      }
      frame "Macro: Exit" {
        # "Exit Macro\n(This is called once, when the VI exits)"
        n109 = Unbundle By Name(w284) -> ("Core.Close Panel on Exit?"=w283:bool)
        n110 = Select(t="UI: Front Panel State >> Close", s=w283, f="") -> (s? t:f=w280:string)
        n111 = call <vilib>:"Add State(s) to Queue__jki_lib_state_machine.vi"("State(s) in (\"\")"=w280, "State(s) at Back (\"\")"="Data: Cleanup\nExit") -> ("States Out"=w278:string)  [unwired: 13 in]
        n112 = call <vilib>:"Add State(s) to Queue__jki_lib_state_machine.vi"("State(s) in Front (\"\")"=w278, "State(s) in (\"\")"=w287) -> ("States Out"=w286:string)  [unwired: 13 in]
      }
      frame "---------- New Category ----------" {
        # "Template Separator\n(You can make a copy of, or modify, this frame)"
        n113 = call <vilib>:"Add State(s) to Queue__jki_lib_state_machine.vi"("State(s) in (\"\")"=w291) -> ("States Out"=w290:string)  [unwired: 14 in]
      }
      frame "Action: Plot data" {
        n114 = Unbundle By Name(w299) -> ("Graph parameters.Timestamp"=w316:dbl[], "Graph parameters.variable 1"=w315:dbl[], "Graph parameters.variable 2"=w314:dbl[], "Graph parameters.variable 3"=w313:dbl[], "Graph parameters.variable 7"=w312:dbl[], "Graph parameters.variable 8"=w311:dbl[])
        n115 = Get Date/Time In Seconds() -> (seconds since 1Jan1904=w324:timestamp)
        n116 = Array Size(array=w316) -> (size(s)=w326:i32)
        n117 = To Double Precision Float(number=w324) -> (double precision float=w322:dbl)
        n118 = Greater?(x=w326, y=14400) -> (0:w323:bool)
        n119 = Bundle("channel 1::2"="channel 1::2", "channel 2::2"="channel 2::2") -> (→"XY Graph 5":T2)  [unwired: 1 in]
        n120 = case shown="True" w323 {
          tunnel: w322 -> [w347 w372]
          tunnel: "reading.var 1::1" -> [w336 w367]
          tunnel: "reading.var 2::1" -> [w346 w371]
          tunnel: "reading.var 3::1" -> [w337 w368]
          tunnel: "reading.var 6::1" -> [w345 w370]
          tunnel: "reading.var 7::1" -> [w344 w369]
          tunnel: [w343 w353] -> w297
          tunnel: [w342 w352] -> w296
          tunnel: [w341 w351] -> w295
          tunnel: [w340 w350] -> w294
          tunnel: [w339 w349] -> w293
          tunnel: [w338 w348] -> w292
          tunnel: w316 -> [w335 w366]
          tunnel: w311 -> [w334 w365]
          tunnel: w312 -> [w333 w364]
          tunnel: w313 -> [w332 w363]
          tunnel: w314 -> [w331 w362]
          tunnel: w315 -> [w330 w361]
          frame False {
            n121 = Build Array (concatenate)(w335, w347) -> (w343:dbl[])
            n122 = Build Array (concatenate)(w330, w336) -> (w342:dbl[])
            n123 = Build Array (concatenate)(w331, w346) -> (w341:dbl[])
            n124 = Build Array (concatenate)(w332, w337) -> (w340:dbl[])
            n125 = Build Array (concatenate)(w333, w345) -> (w339:dbl[])
            n126 = Build Array (concatenate)(w334, w344) -> (w338:dbl[])
          }
          frame True {
            w360 = 0
            n127 = Build Array (concatenate)(w366, w372) -> (w359:dbl[])
            n128 = Build Array (concatenate)(w361, w367) -> (w358:dbl[])
            n129 = Build Array (concatenate)(w362, w371) -> (w357:dbl[])
            n130 = Build Array (concatenate)(w363, w368) -> (w356:dbl[])
            n131 = Build Array (concatenate)(w364, w370) -> (w355:dbl[])
            n132 = Build Array (concatenate)(w365, w369) -> (w354:dbl[])
            n133 = Delete From Array(array=w359, index=w360) -> (array with subset deleted=w353:dbl[])  [unwired: 1 in, 1 out]
            n134 = Delete From Array(array=w358, index=w360) -> (array with subset deleted=w352:dbl[])  [unwired: 1 in, 1 out]
            n135 = Delete From Array(array=w357, index=w360) -> (array with subset deleted=w351:dbl[])  [unwired: 1 in, 1 out]
            n136 = Delete From Array(array=w356, index=w360) -> (array with subset deleted=w350:dbl[])  [unwired: 1 in, 1 out]
            n137 = Delete From Array(array=w355, index=w360) -> (array with subset deleted=w349:dbl[])  [unwired: 1 in, 1 out]
            n138 = Delete From Array(array=w354, index=w360) -> (array with subset deleted=w348:dbl[])  [unwired: 1 in, 1 out]
          }
        }
        n139 = To Time Stamp(1:w297) -> (0:w303:timestamp[])
        n140 = Bundle(w303, w295) -> (w306:cluster{timestamp[], dbl[]})  [unwired: 1 in]
        n141 = Bundle(w303, w294) -> (w305:cluster{timestamp[], dbl[]})  [unwired: 1 in]
        n142 = Bundle(w303, w293) -> (w302:cluster{timestamp[], dbl[]})  [unwired: 1 in]
        n143 = Bundle(w303, w292) -> (w301:cluster{timestamp[], dbl[]})  [unwired: 1 in]
        n144 = Build Array(w306, w305) -> (→"XY Graph 2":cluster{timestamp[], dbl[]}[])
        n145 = Build Array(w302, w301) -> (→"XY Graph 3":cluster{timestamp[], dbl[]}[])
        n146 = Bundle(w303, w296) -> (→"XY Graph":cluster{timestamp[], dbl[]})  [unwired: 1 in]
        n147 = call <vilib>:"Add State(s) to Queue__jki_lib_state_machine.vi"("State(s) in (\"\")"=w329) -> ("States Out"=w328:string)  [unwired: 14 in]
        n148 = Bundle By Name(cluster=w299, "Graph parameters.Timestamp"=w297, "Graph parameters.variable 1"=w296, "Graph parameters.variable 2"=w295, "Graph parameters.variable 3"=w294, "Graph parameters.variable 7"=w293, "Graph parameters.variable 8"=w292) -> (w298:T6)
      }
      frame "New Category: 2" {
        # "Your code here.\n(You can make a copy of, or modify, this frame)"
        n149 = call <vilib>:"Add State(s) to Queue__jki_lib_state_machine.vi"("State(s) in (\"\")"=w376) -> ("States Out"=w375:string)  [unwired: 14 in]
      }
    }
  }
